vi "Read Double.vi"(8 "error in (no error)":errorcluster, 11 "VISA resource name":refnum<visa-resource-name>) -> (0 "error out":errorcluster, 2 "Double":dbl, 3 "VISA resource name out":refnum<visa-resource-name>)   [LabVIEW 2015]
panel:
  out "read buffer":string
  out "return count":u32
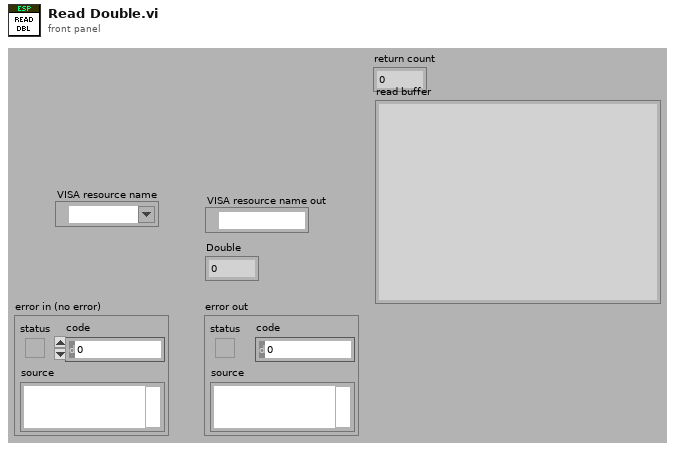
[diagram p1: front panel]
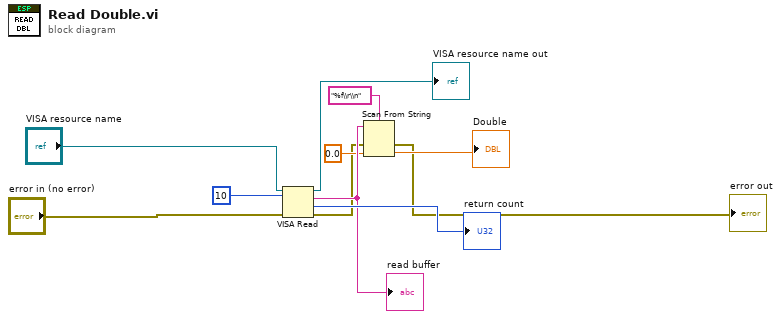
[diagram p0: block diagram]
diagram:
  n1 = VISA Read(VISA resource name="VISA resource name", byte count=u32 10, error in (no error)="error in (no error)") -> (VISA resource name out=→"VISA resource name out":refnum<visa-resource-name>, read buffer=w6:string, return count=→"return count":u32, error out=w2:errorcluster)
  "read buffer" <- w6
  n2 = Scan From String(format string="%f\\r\\n", input string=w6, error in=w2, default 1=0.0) -> (error out=→"error out":errorcluster, output 1=→"Double":dbl)  [unwired: 1 in, 2 out]
